vi "Show Waveform Chart.vi"(2 "stop":bool, 3 "waveform chart":cluster{dbl, i32}(graph)={0.5489327770964688, 0}) -> ()   [LabVIEW 2011]
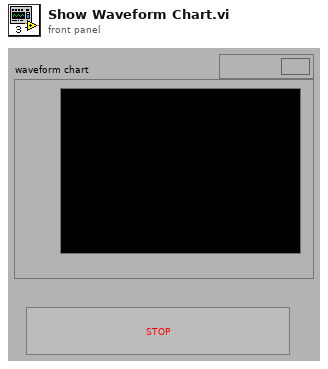
[diagram p1: front panel]
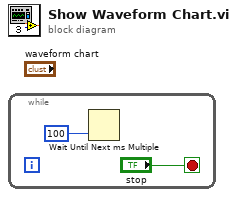
[diagram p0: block diagram]
diagram:
  n1 = while {
    stop <- "stop" stop-if-true
    n2 = Wait Until Next ms Multiple(millisecond multiple=u32 100) -> ()  [unwired: 1 out]
  }
